vi "writeToXML.vi"(8 "error in (no error)":errorcluster, 10 "classLabel":string, 11 "DifftrackRADec in":refnum<class "DifftrackRADec.lvclass">) -> (0 "error out":errorcluster, 2 "XML out":string, 3 "DifftrackRADec out":refnum<class "DifftrackRADec.lvclass">)   [LabVIEW 2022 SP3, in "TCSDataDefinitions.lvlib" / "TCSCommand.lvlib" / "TargetConfiguration.lvlib" / "Target.lvlib" / "DifftrackRADec.lvclass"]
uses:
  DifftrackRADec.lvclass
  <userlib>/Common/UnitsAndXML/FlattenItemWithUnitToXML/FlattenAngularVelocityToXML/AngularVelocityUnit.ctl
  DifftrackRADec.lvclass/DifftrackRADec.ctl
  Difftrack.lvclass
  <userlib>/Common/UnitsAndXML/UnitsAndXML.lvlib
  <userlib>/Common/XML/XMLGenerator/XMLGenerator.lvclass
  <userlib>/Common/XML/XMLAttributeGenerator/XMLAttributeGenerator.lvclass
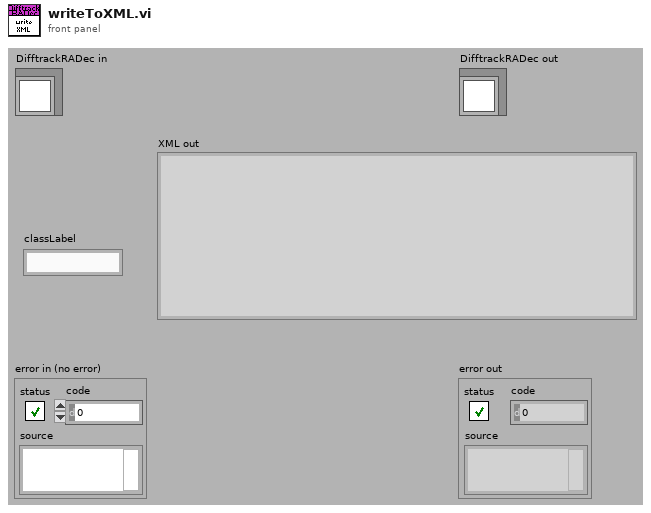
[diagram p1: front panel]
types:
  T1 = typedef "UnitsAndXML.lvlib/AngularVelocityUnit.ctl" = enum16{"\"/a", "deg/s", "\"/s"}
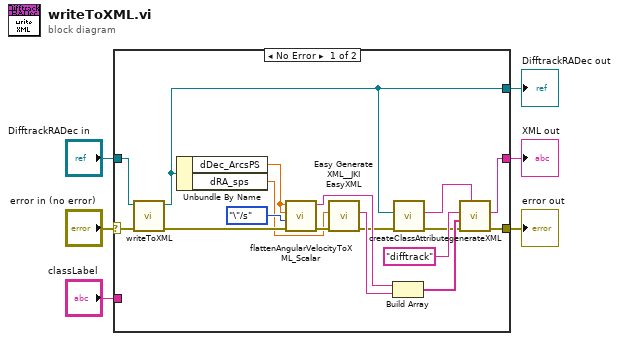
[diagram p0: block diagram]
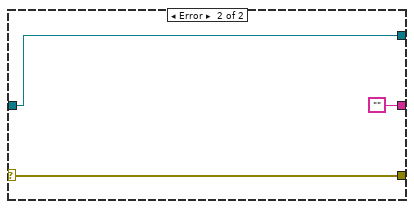
[diagram p2: hidden frame]
diagram:
  n1 = case shown="No Error" "error in (no error)" {
    selector: "error in (no error)" -> [w18 w26]
    tunnel: [w17 w26] -> w5
    tunnel: [w8 w25] -> w3
    tunnel: "DifftrackRADec in" -> [w23 w25]
    tunnel: "classLabel" -> [_ _]
    tunnel: [w11 ""] -> w1
    frame No Error {
      n2 = call-parent "writeToXML.vi"("error in (no error)"=w18, "Difftrack in"=w23) -> ("error out"=w20:errorcluster, "Difftrack out"=w8:refnum<class "DifftrackRADec.lvclass">)  [unwired: 7 in, 1 out]
      n3 = Unbundle By Name(w8) -> ("dDec_ArcsPS"=w22:dbl[unit], "dRA_sps"=w14:dbl)
      n4 = call <userlib>:"flattenAngularVelocityToXML_Scalar.vi"("error in (no error)"=w20, "angularVelocityUnitInXML"=AngularVelocityUnit."\"/s", "anuglarVelocityAgain"=w22, "angularVelocity"=w22) -> ("error out"=w19:errorcluster, "xmlString"=w16:string)  [unwired: 6 in]
      n5 = call <vilib>:"Easy Generate XML__JKI EasyXML.vi"("error in (no error)"=w19, "LabVIEW Data"=w14) -> ("error out"=w7:errorcluster, "XML String"=w15:string)  [unwired: 8 in]
      n6 = Build Array(w16, w15) -> (w13:string[])
      n7 = call <userlib>:"createClassAttribute.vi"("error in (no error)"=w7, "LVClass In"=w8) -> ("error out"=w9:errorcluster, "AttributeString"=w10:string)  [unwired: 7 in, 1 out]
      n8 = call <userlib>:"generateXML.vi"("attributeString"=w10, "error in"=w9, "childrenXML"=w13, "elementName"="difftrack" ("Class Label")) -> ("error out"=w17:errorcluster, "XML out"=w11:string)  [unwired: 5 in, 1 out]
    }
    frame Error {
    }
  }
  "error out" <- w5
  "DifftrackRADec out" <- w3
  "XML out" <- w1
